vi "From BananaLeaf.TestCase.vi"(11 "Leaf.Properties.TestCase":refnum<class "Leaf.Properties.Test.lvclass">) -> (2 "Properties.Test":refnum<class "Properties.Test.lvclass">)   [LabVIEW 2021, in "Banana.Caraya.lvlib" / "Leaf.Properties.Test.lvclass"]
uses:
  Leaf.Properties.Test.lvclass
  C:/Repositories/LVOS/Bananas/lv-src/Banana.Caraya/Leaf.Properties/Leaf.Properties.lvclass
  Leaf.Properties/Leaf.Properties.lvclass/Leaf.Properties.ctl
  Leaf.Properties.Test.lvclass/Leaf.Properties.Test.ctl
  Leaf.Properties/Leaf.Properties.lvclass
  <vilib>/addons/_JKI Toolkits/Caraya/classes/Properties.Test/Properties.Test.lvclass
  C:/Program Files (x86)/National Instruments/LabVIEW 2021/vi.lib/addons/_JKI Toolkits/Caraya/classes/Properties/Properties.lvclass
  C:/Repositories/LVOS/Bananas/lv-src/Bananas/Leaf/Leaf.lvclass
  C:/Repositories/LVOS/Bananas/lv-src/Bananas/Leaf.TestCase/Leaf.TestCase.lvclass
  C:/Repositories/LVOS/Bananas/lv-src/Banana.Caraya/Leaf.Properties.Test/Leaf.Properties.Test.lvclass
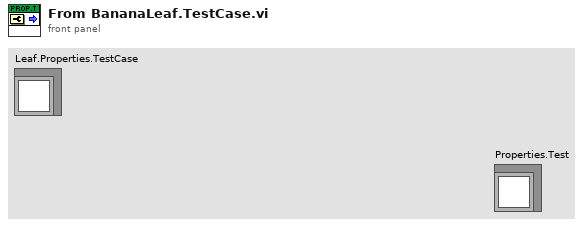
[diagram p1: front panel]
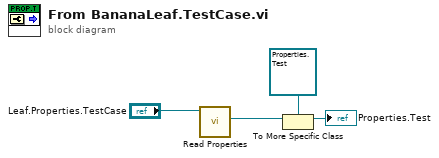
[diagram p0: block diagram]
diagram:
  n1 = call "Read Properties.vi"("Leaf.Properties in"="Leaf.Properties.TestCase") -> ("Properties"=w3:refnum<class "Properties.lvclass">)  [unwired: 9 in, 1 out]
  n2 = To More Specific Class(target class=refnum<class "Properties.Test.lvclass"> refnum ("Properties.Test"), reference=w3) -> (specific class reference=→"Properties.Test":refnum<class "Properties.Test.lvclass">)  [unwired: 1 in, 1 out]
